vi "DumbDash Get Control Type.vi"(10 "reference":refnum<vi>) -> (2 "Type":T1)   [LabVIEW 2014]
uses:
  DumbDash Control Type.ctl
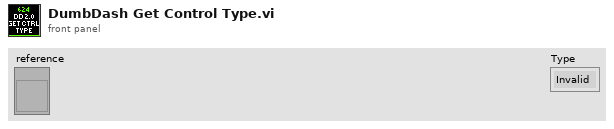
[diagram p1: front panel]
types:
  T1 = typedef "DumbDash Control Type.ctl" = enum16{"Invalid", "Number", "Boolean", "String"}
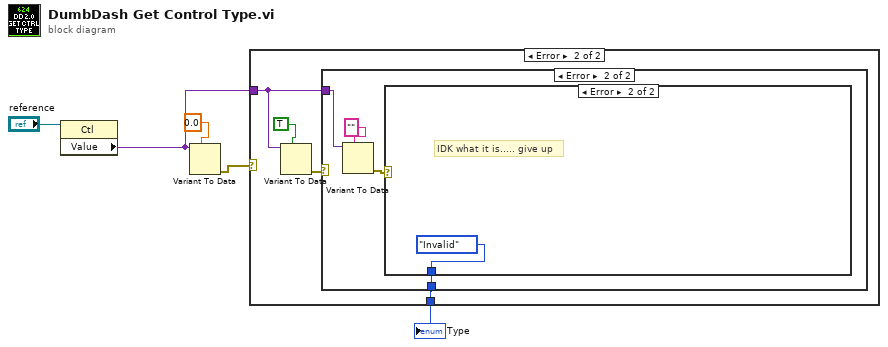
[diagram p0: block diagram]
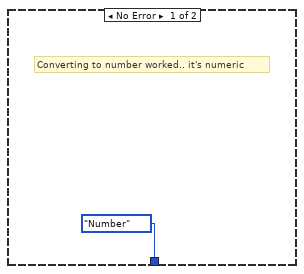
[diagram p2: hidden frame]
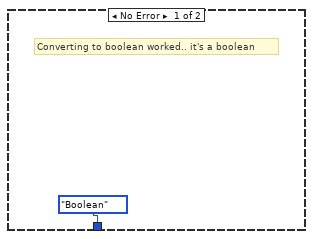
[diagram p3: hidden frame]
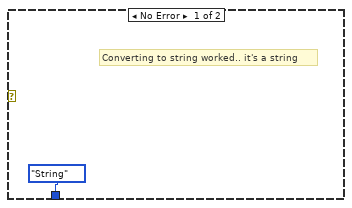
[diagram p4: hidden frame]
diagram:
  n1 = property class="Ctl"(reference="reference") -> ("Value"=w3:variant)  [unwired: 1 in, 2 out]
  n2 = Variant To Data(type=0.0, Variant=w3) -> (error out=w4:errorcluster)  [unwired: 1 in, 1 out]
  n3 = case shown="Error" w4 {
    tunnel: w3 -> [_ w8]
    tunnel: [DumbDash_Control_Type."Number" w7] -> w1
    frame No Error {
      # "Converting to number worked.. it's numeric"
    }
    frame Error {
      n4 = Variant To Data(type=TRUE, Variant=w8) -> (error out=w9:errorcluster)  [unwired: 1 in, 1 out]
      n5 = case shown="Error" w9 {
        tunnel: w8 -> [_ w15]
        tunnel: [DumbDash_Control_Type."Boolean" w12] -> w7
        frame No Error {
          # "Converting to boolean worked.. it's a boolean"
        }
        frame Error {
          n6 = Variant To Data(type="", Variant=w15) -> (error out=w13:errorcluster)  [unwired: 1 in, 1 out]
          n7 = case shown="Error" w13 {
            tunnel: [DumbDash_Control_Type."String" DumbDash_Control_Type."Invalid"] -> w12
            frame No Error {
              # "Converting to string worked.. it's a string"
            }
            frame Error {
              # "IDK what it is..... give up"
            }
          }
        }
      }
    }
  }
  "Type" <- w1
